vi "PTScanner.check steps conditions.vi"(0 "i ref in":refnum<vi>, 5 "error in (no error)":errorcluster) -> (14 "i ref out":refnum<vi>, 16 "Finished":bool, 17 "All Finished":bool, 19 "error out":errorcluster)   [LabVIEW 2014, in "PTScanner.lvlib"]
uses:
  PTScanner.lvlib
  CSlibraries-extern/DimLVEvent/LVDimInterface/LVDimInterface.lvlib
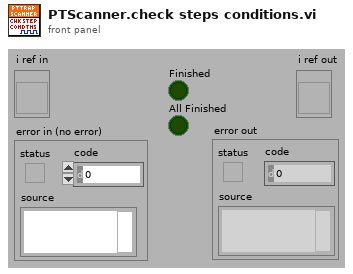
[diagram p1: front panel]
types:
  T1 = typedef "PTScanner.lvlib/PTScanner.i attribute.ctl" = cluster{"Object cmds":T2[], "Steps":cluster{"Finished":bool, "cmd setup":T3[]}[], "curStep":i32, "DIM IDs":cluster{"AllFinished":i32, "Finished":i32, "curStep":i32, "nofSteps":i32, "NomValues":i32[], "1D-Min":i32, "1D-Max":i32, "Dimensions":i32, "MaxDimensions":i32, "ScanedDeviceNames":i32[]}, "All Finished":bool, "DIMs in use":string[], "Running":bool, "Scan Delay":u32, "loop":bool, "Paused":bool, "Formed":bool}
  T2 = typedef "PTScanner.lvlib/PTScanner.obj parameters.ctl" = cluster{"object":string, "DIM address":string, "method":string, "data descriptor":string, "method parameters":cluster{"Name":string, "Descr":string, "Value":string, "Value?":bool}[], "Call Mode":enum16{"Simple DIM", "Synchronous"}, "actValue":dbl, "Centroid":dbl, "Minus Delta":dbl, "Plus Delta":dbl, "increment":dbl, "DIM Status":cluster{"no link":bool, "quality":i32, "Time Stamp":timestamp}, "range":dbl, "DIMChannelIndex":i32}
  T3 = typedef "PTScanner.lvlib/PTScanner.step obj parameters.ctl" = cluster{"obj index":i32, "nomValue":dbl, "fulfilled":bool}
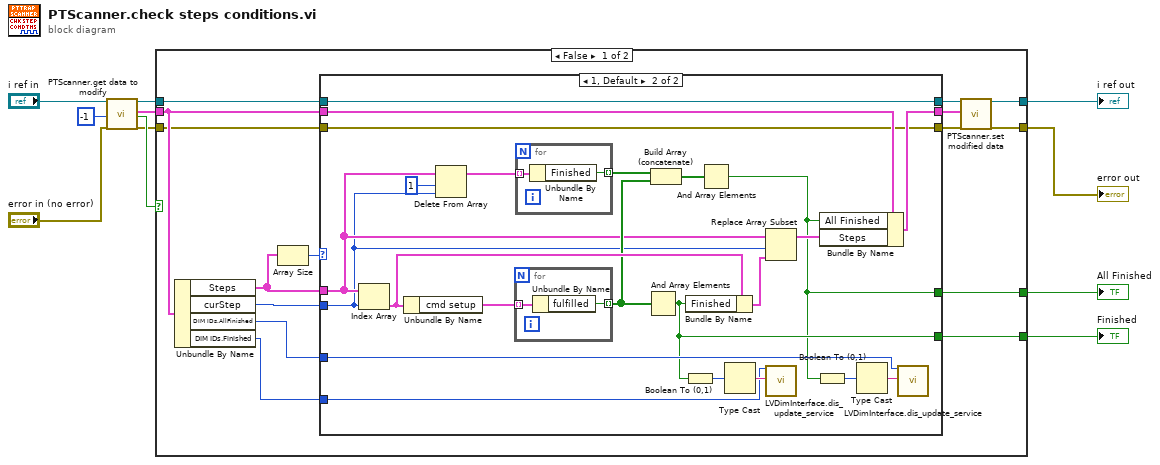
[diagram p0: block diagram]
diagram:
  n1 = call "PTScanner.get data to modify.vi"("i ref in"="i ref in", "ms timeout (10000)"=-1, "error in (no error)"="error in (no error)") -> ("i ref out"=w10:refnum<vi>, "i attribute"=w11:T1, "timed out"=w9:bool, "error out"=w7:errorcluster)  [unwired: 13 in]
  n2 = case shown="False" w9 {
    tunnel: w11 -> [w26 _]
    tunnel: w10 -> [w17 w58]
    tunnel: w7 -> [w15 w57]
    tunnel: [w24 w58] -> w4
    tunnel: [w23 w57] -> w3
    tunnel: [w13 _] -> w2
    tunnel: [w12 _] -> w1
    frame False {
      n3 = Unbundle By Name(w26) -> ("Steps"=w21:cluster{"Finished":bool, "cmd setup":T3[]}[], "curStep"=w22:i32, "DIM IDs.AllFinished"=w18:i32, "DIM IDs.Finished"=w19:i32)
      n4 = Array Size(array=w21) -> (size(s)=w20:i32)
      n5 = case shown="1, Default" w20 {
        tunnel: w26 -> [w29 w45]
        tunnel: [w29 w42] -> w25
        tunnel: w21 -> [_ w41]
        tunnel: w22 -> [_ w40]
        tunnel: w19 -> [_ w37]
        tunnel: w18 -> [_ w34]
        tunnel: w17 -> [w28 w33]
        tunnel: [w28 w33] -> w16
        tunnel: w15 -> [w27 w32]
        tunnel: [w27 w32] -> w14
        tunnel: [_ w31] -> w13
        tunnel: [_ w30] -> w12
        frame 0 {
        }
        frame 1, Default {
          n6 = Index Array(array=w41, index=w40) -> (element=w51:cluster{"Finished":bool, "cmd setup":T3[]})
          n7 = Unbundle By Name(w51) -> ("cmd setup"=w52:T3[])
          n8 = Delete From Array(array=w41, length=1, index=w40) -> (array with subset deleted=w49:cluster{"Finished":bool, "cmd setup":T3[]}[])  [unwired: 1 out]
          n9 = for {
            tunnel: w52 -> [w56] mode=indexing
            tunnel: [w55] -> w47 mode=indexing
            n10 = Unbundle By Name(w56) -> ("fulfilled"=w55:bool)
          }
          n11 = for {
            tunnel: w49 -> [w54] mode=indexing
            tunnel: [w53] -> w48 mode=indexing
            n12 = Unbundle By Name(w54) -> ("Finished"=w53:bool)
          }
          n13 = And Array Elements(Boolean array=w47) -> (logical AND=w31:bool)
          n14 = Build Array (concatenate)(w48, w47) -> (w46:bool[])
          n15 = Boolean To (0,1)(Boolean=w31) -> (0, 1=w38:i16)
          n16 = Bundle By Name(cluster=w51, "Finished"=w31) -> (w44:cluster{"Finished":bool, "cmd setup":T3[]})
          n17 = And Array Elements(Boolean array=w46) -> (logical AND=w30:bool)
          n18 = Type Cast(x=w38) -> (*(type *) &x=w39:string)  [unwired: 1 in]
          n19 = Replace Array Subset(array=w41, new element=w44, index=w40) -> (w43:cluster{"Finished":bool, "cmd setup":T3[]}[])
          n20 = call "LVDimInterface.dis_update_service.vi"("my_serviceID"=w37, "data"=w39) -> ()  [unwired: 15 in, 3 out]
          n21 = Boolean To (0,1)(Boolean=w30) -> (0, 1=w35:i16)
          n22 = Bundle By Name(cluster=w45, "All Finished"=w30, "Steps"=w43) -> (w42:T1)
          n23 = Type Cast(x=w35) -> (*(type *) &x=w36:string)  [unwired: 1 in]
          n24 = call "LVDimInterface.dis_update_service.vi"("my_serviceID"=w34, "data"=w36) -> ()  [unwired: 15 in, 3 out]
        }
      }
      n25 = call "PTScanner.set modified data.vi"("i ref in"=w16, "CLASS.i attribute"=w25, "error in (no error)"=w14) -> ("i ref out"=w24:refnum<vi>, "error out"=w23:errorcluster)  [unwired: 15 in]
    }
    frame True {
    }
  }
  "i ref out" <- w4
  "error out" <- w3
  "Finished" <- w2
  "All Finished" <- w1
